vi "Write Active.vi"(8 "error in (no error)":errorcluster, 10 "Active":bool, 11 "Integrator in":refnum<class "Integrator.lvclass">) -> (0 "error out":errorcluster, 3 "Integrator out":refnum<class "Integrator.lvclass">)   [LabVIEW 2016, in "Integrator.lvclass"]
uses:
  Integrator.lvclass
  Integrator.lvclass/Integrator.ctl
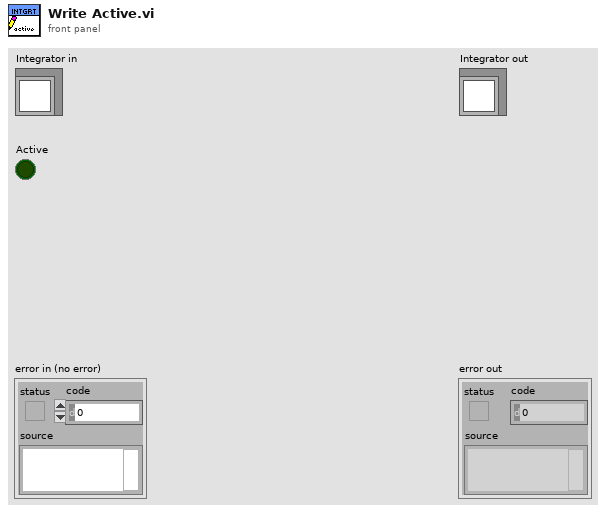
[diagram p1: front panel]
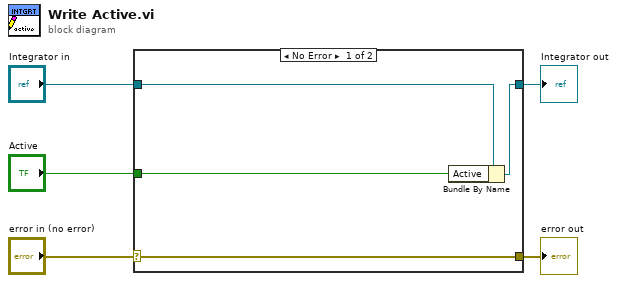
[diagram p0: block diagram]
diagram:
  n1 = case shown="No Error" "error in (no error)" {
    selector: "error in (no error)" -> [w9 w10]
    tunnel: [w9 w10] -> w4
    tunnel: [w7 w11] -> w2
    tunnel: "Integrator in" -> [w8 w11]
    tunnel: "Active" -> [w6 _]
    frame No Error {
      n2 = Bundle By Name(cluster=w8, "Active"=w6) -> (w7:refnum<class "Integrator.lvclass">)
    }
    frame Error {
    }
  }
  "error out" <- w4
  "Integrator out" <- w2
